vi "Dashboard Main.vi"() -> ()   [LabVIEW 2016]
uses:
  <vilib>/Utility/miscctls.llb/LVRowAndColumnTypeDef.ctl
  <vilib>/event_ctls.llb/eventvkey.ctl
  <vilib>/Rock Robotics/Network Tables/NT Read Numeric Array.vi
  <vilib>/Rock Robotics/Network Tables/NT Read Boolean.vi
  <vilib>/Rock Robotics/WPI/Dashboard/WPI_DashboardLogging Global.vi
panel:
  in  "Camera Settings Right":T1={"Frame Rate"=30, "Compression"=30, "Size"=1, "DB Camera Config"=FALSE} {"Frame Rate" scale=1.0..30.0; "Compression" scale=100.0..-1.0; "Size" items=["640x480", "320x240", "160x120"]}
  out "Camera Info":cluster{"Mbps LED":bool, "Mbps":dbl, "fps":dbl} {"fps" format="%#.1g"; "Mbps" format="%#.1g"}
  in  "Camera Settings":T1={"Frame Rate"=30, "Compression"=30, "Size"=1, "DB Camera Config"=FALSE} {"Frame Rate" scale=1.0..30.0; "Compression" scale=100.0..-1.0; "Size" items=["640x480", "320x240", "160x120"]}
  in  "TCP":refnum<k5>
  in  "Rec Mode":enum32{"Stop", "Record", "Playback"}(radio)
  out "Robot IP":string
  out "Image Message":string="Timeout in Camera Communications"
  in  "Dashboard Tab":T2(tab)
  in  "Select Auto":string(combo)="Select Autonomous ..."
  out "NT Connection":bool
  out "MotorChart R":cluster{"Numeric":dbl, "Numeric":dbl}(graph)
  out "MotorChart L":cluster{"Numeric":dbl, "Numeric":dbl}(graph)
  out "MotorSliders R":cluster{"MotorSlide1":dbl, "MotorSlide2":dbl} {"MotorSlide2" scale=-1.0..1.0 scale format="%#_2e"; "MotorSlide1" scale=-1.0..1.0 scale format="%#_2e"}
  out "MotorSliders L":cluster{"MotorSlide1":dbl, "MotorSlide2":dbl} {"MotorSlide2" scale=-1.0..1.0 scale format="%#_2e"; "MotorSlide1" scale=-1.0..1.0 scale format="%#_2e"}
  out "Gyro":dbl(knob) scale=0.0..360.0
  out "JS1 Z":dbl(slide) scale=-1.0..1.0 scale format="%#_2e"
  out "JS1 Graph":cluster{"X":dbl, "Y":dbl}[](graph)
  out "JS1 Buttons":T3
  out "JS2 Z":dbl(slide) scale=-1.0..1.0 scale format="%#_2e"
  out "JS2 Graph":cluster{"X":dbl, "Y":dbl}[](graph)
  out "JS2 Buttons":T3
  out "Mode":T4(ring)=enum."Auto Disabled"
  out "Camera Image Right":T5(plugin-control)
  in  "ACTION":u16(ring) items=["Place Gear (Default)", "Cross Line Only", "Place Gear And Cross Line"]
  in  "POSITION":dbl format="%#_3f"
  in  "Left":dbl
  in  "Motor":dbl
  in  "Right":dbl
  in  "Camera Name":string(combo)="No Camera Selection"
  out "Scaling Mode":bool
  in  "Camera Name Right":string(combo)="No Camera Selection"
  in  "Test Slider":dbl(slide) scale=0.0..100.0 scale format="%#_3g"
  in  "On/Off":bool caption="Solenoid"
  in  "Test Name":u16(ring) items=["Select the test to run..."]
  in  "Test Tree":string(tree)
  in  "Motor":cluster{"Value":dbl, "Enable":bool} {"Value" scale=-1.0..1.0 scale format="%#_3g"}
  out "Progress":T6 {"Test Progress" scale=0.0..100.0}
  in  "Rev/Fwd":cluster{"Forward":bool, "Reverse":bool}
  in  "Test Ring":u16(ring) items=["Monochrome", "Color"]
  out "Cmd Status":string
  in  "Execute Command":bool
  in  "Command Params":string[][](table)
  in  "Command Selection":i32(listbox)
  in  "CheckList":i32(listbox)
  out "Tree":string(tree)
  out "Camera Image":T5(plugin-control)
  out "Background":bool
  # "HW"
  # "HW"
  # "Joysticks"
  # "Drive Motors"
  # "Front"
  # "Right"
  # "Left"
  # "Back"
  # "AUTONOMOUS- FILL OUT BEFORE EVERY MATCH"
  # "Supply a number between 1 and 3"
  # "Select an action"
  # "Flywheel Speed"
  # "Carousel Motor"
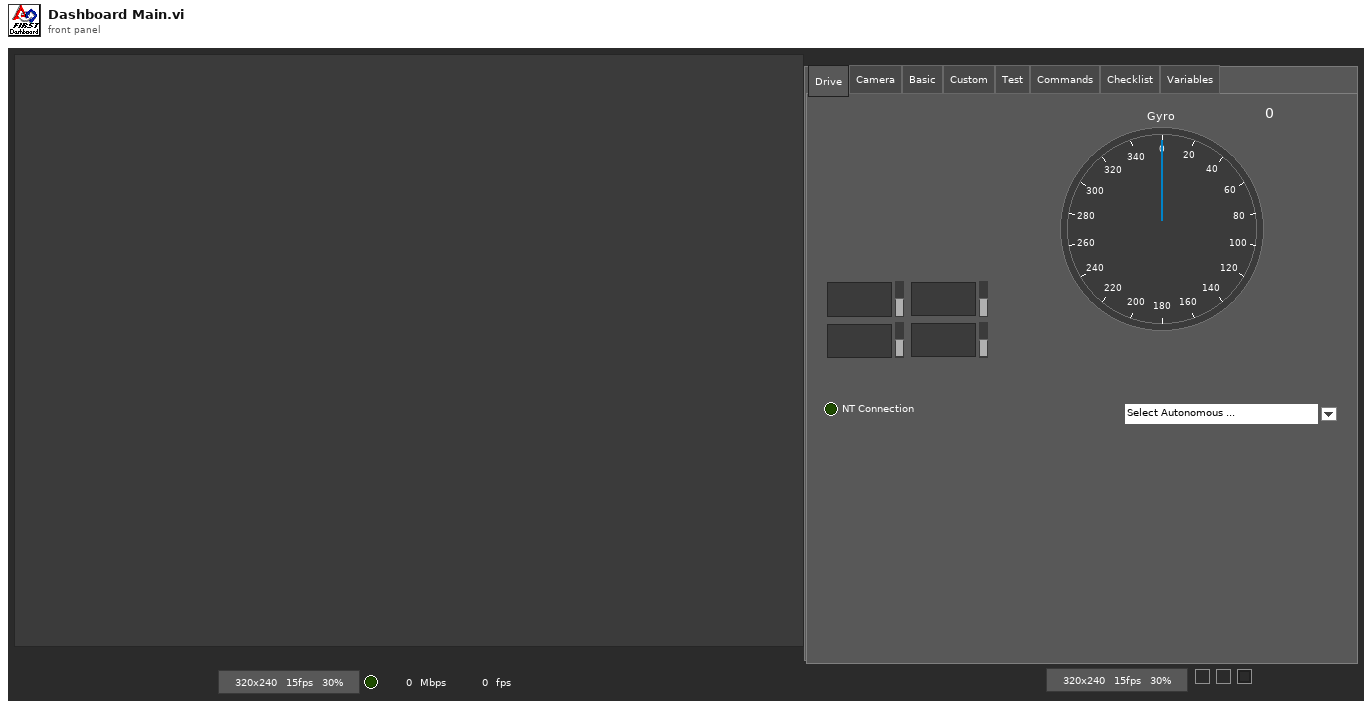
[diagram p1: front panel]
types:
  T1 = cluster{"Frame Rate":i32, "Compression":i32, "Size":u16, "DB Camera Config":bool}
  T2 = enum32{"Drive", "Camera", "Basic", "Custom", "Test", "Commands", "Checklist", "Variables"}
  T3 = cluster{bool, bool, bool, bool, bool, bool, bool, bool, bool, bool, bool, bool}
  T4 = enum8{"Tele-Op Disabled", "Tele-Op Enabled", "Auto Disabled", "Auto Enabled", "Test Disabled", "Test Enabled", "Disconnected", "No Code", "E-Stop"}
  T5 = typedef "IMAQ Image.ctl" = refnum<image>
  T6 = cluster{"Test Progress":u8, "Test Progress Text":string}
  T7 = typedef "Image Type" = u32
  T8 = cluster{"IDs":cluster{"RPC field ID":u16, "Unique ID":u16}, "String":string}
  T9 = enum32{"Drive", "Basic", "Custom", "Test", "Checklist", "Variables"}
  T10 = cluster{"Camera Streams":i32, cluster{"occurrence":refnum<k4>, "New Image":T5}[]}
  T11 = cluster{"Error Strings":string, "Disable Counts":cluster{u16, u16}, "Rail Faults":cluster{u16, u16, u16}, "Robot IP":string, "DB Mode":u8, "Event Info":cluster{"Name":string, "Type":u8, "Number":u16, "Replay":u8}}
  T12 = cluster{"Storage":cluster{"Disk Free":u64, "RAM Block":u32, "RAM free":u32}, "CPU Utilization":cluster{"CPU % ISR":sgl, "CPU % Time Crit":sgl, "CPU % Timed Str":sgl, "CPU % High":sgl, "CPU % Above":sgl, "CPU % Normal":sgl, "CPU % Low":sgl}, "CAN":cluster{"% Bus Utilization":sgl, "Bus Off Cnt":u32, "TX_FIFO Full Cnt":u32, "Receive Error Cnt":u8, "Transmit Error Cnt":u8}, "HID":cluster{"HID Outputs":u32, "Rumble Low":u16, "Rumble High":u16}[]}
  T13 = cluster{"Status bits":cluster{"Test Mode":bool, "Autonomous":bool, "Enabled":bool, "Code Start":bool, "Brownout":bool, "Reserved 2":bool, "Reserved 3":bool, "E-Stop":bool}, "Code Trace":cluster{"Disabled":bool, "TeleOp":bool, "Auto":bool, "Test":bool}, "Controller Type":enum16{"unknown", "cRIO", "roboRio"}, "Code?":enum16{"unknown", "noCode", "code"}, "Battery V":dbl}
  T14 = cluster{"Control Bits":cluster{"TestMode":bool, "Autonomous":bool, "Enabled":bool, "FMS Present":bool, bool, bool, bool, "E-Stop":bool}, "Team Station ":u8, "Countdown":sgl, "Joystick Values":cluster{"Axes":dbl[], "Buttons":bool[], "POVs":i16[]}[]}
  T15 = cluster{"Axes":dbl[], "Buttons":bool[], "POVs":i16[]}[]
  T16 = cluster{"Axes":dbl[], "Buttons":bool[], "POVs":i16[]}
  T17 = cluster{"Buttons[0]":bool, "Buttons[1]":bool, "Buttons[2]":bool, "Buttons[3]":bool, "Buttons[4]":bool, "Buttons[5]":bool, "Buttons[6]":bool, "Buttons[7]":bool, "Buttons[8]":bool, "Buttons[9]":bool, "Buttons[10]":bool, "Buttons[11]":bool}
  T18 = cluster{"Camera Image":refnum<vi>, "Dashboard Tab":refnum<vi>, "Background":refnum<vi>, "Rec Mode":refnum<vi>, "Test Slider":refnum<vi>, "On/Off ":refnum<vi>, "Test Ring":refnum<vi>, "Rev/Fwd":refnum<vi>, "Test Name":refnum<vi>, "Motor":refnum<vi>, "Progress":refnum<vi>, "CheckList":refnum<vi>, "Tree":refnum<vi>, "Test Tree":refnum<vi>, "Command Params":refnum<vi>, "Command Selection":refnum<vi>, "Execute Command":refnum<vi>, "Cmd Status":refnum<vi>, "Camera Settings":refnum<vi>, "Camera Name":refnum<vi>, "Camera Info":refnum<vi>, "Camera Settings Right":refnum<vi>, "Camera Name Right":refnum<vi>, "Camera Image Right":refnum<vi>}
  T19 = cluster{"Operation":enum16{"Update", "Clear"}, "Color Box":u32}[]
  T20 = typedef "eventvkey.ctl" = enum16{"ASCII", "Enter", "Return", "Shift", "Ctrl", "Alt", "Cmd", "Opt", "Caps", "NumLock", "Clear", "Break", "Up", "Down", "Left", "Right", "Insert", "Delete", "Home", "End", "PageUp", "PageDown", "Escape", "Help", "Pause", "ScrollLock", "F1", "F2", "F3", "F4", "F5", "F6", "F7", "F8", "F9", "F10", "F11", "F12", "F13", "F14", "F15", "F16", "F17", "F18", "F19", "F20", "F21", "F22", "F23", "F24", "Play", "VolumeUp", "VolumeDown", "Mute", "Two Byte Char"}
  T21 = cluster{"Image Size":bool, "Image Type":bool, "Pixel Value":bool, "ROI Information":bool, "Zoom Factor":bool}
  T22 = cluster{"Operation":enum16{"Update", "Clear"}, "Color Box":u32}
  T23 = typedef "LVRowAndColumnTypeDef.ctl" = cluster{"Row":i32, "Column":i32}
  T24 = cluster{"Shift":bool, "Ctrl":bool, "Alt":bool, "Cmd":bool, "Opt":bool}
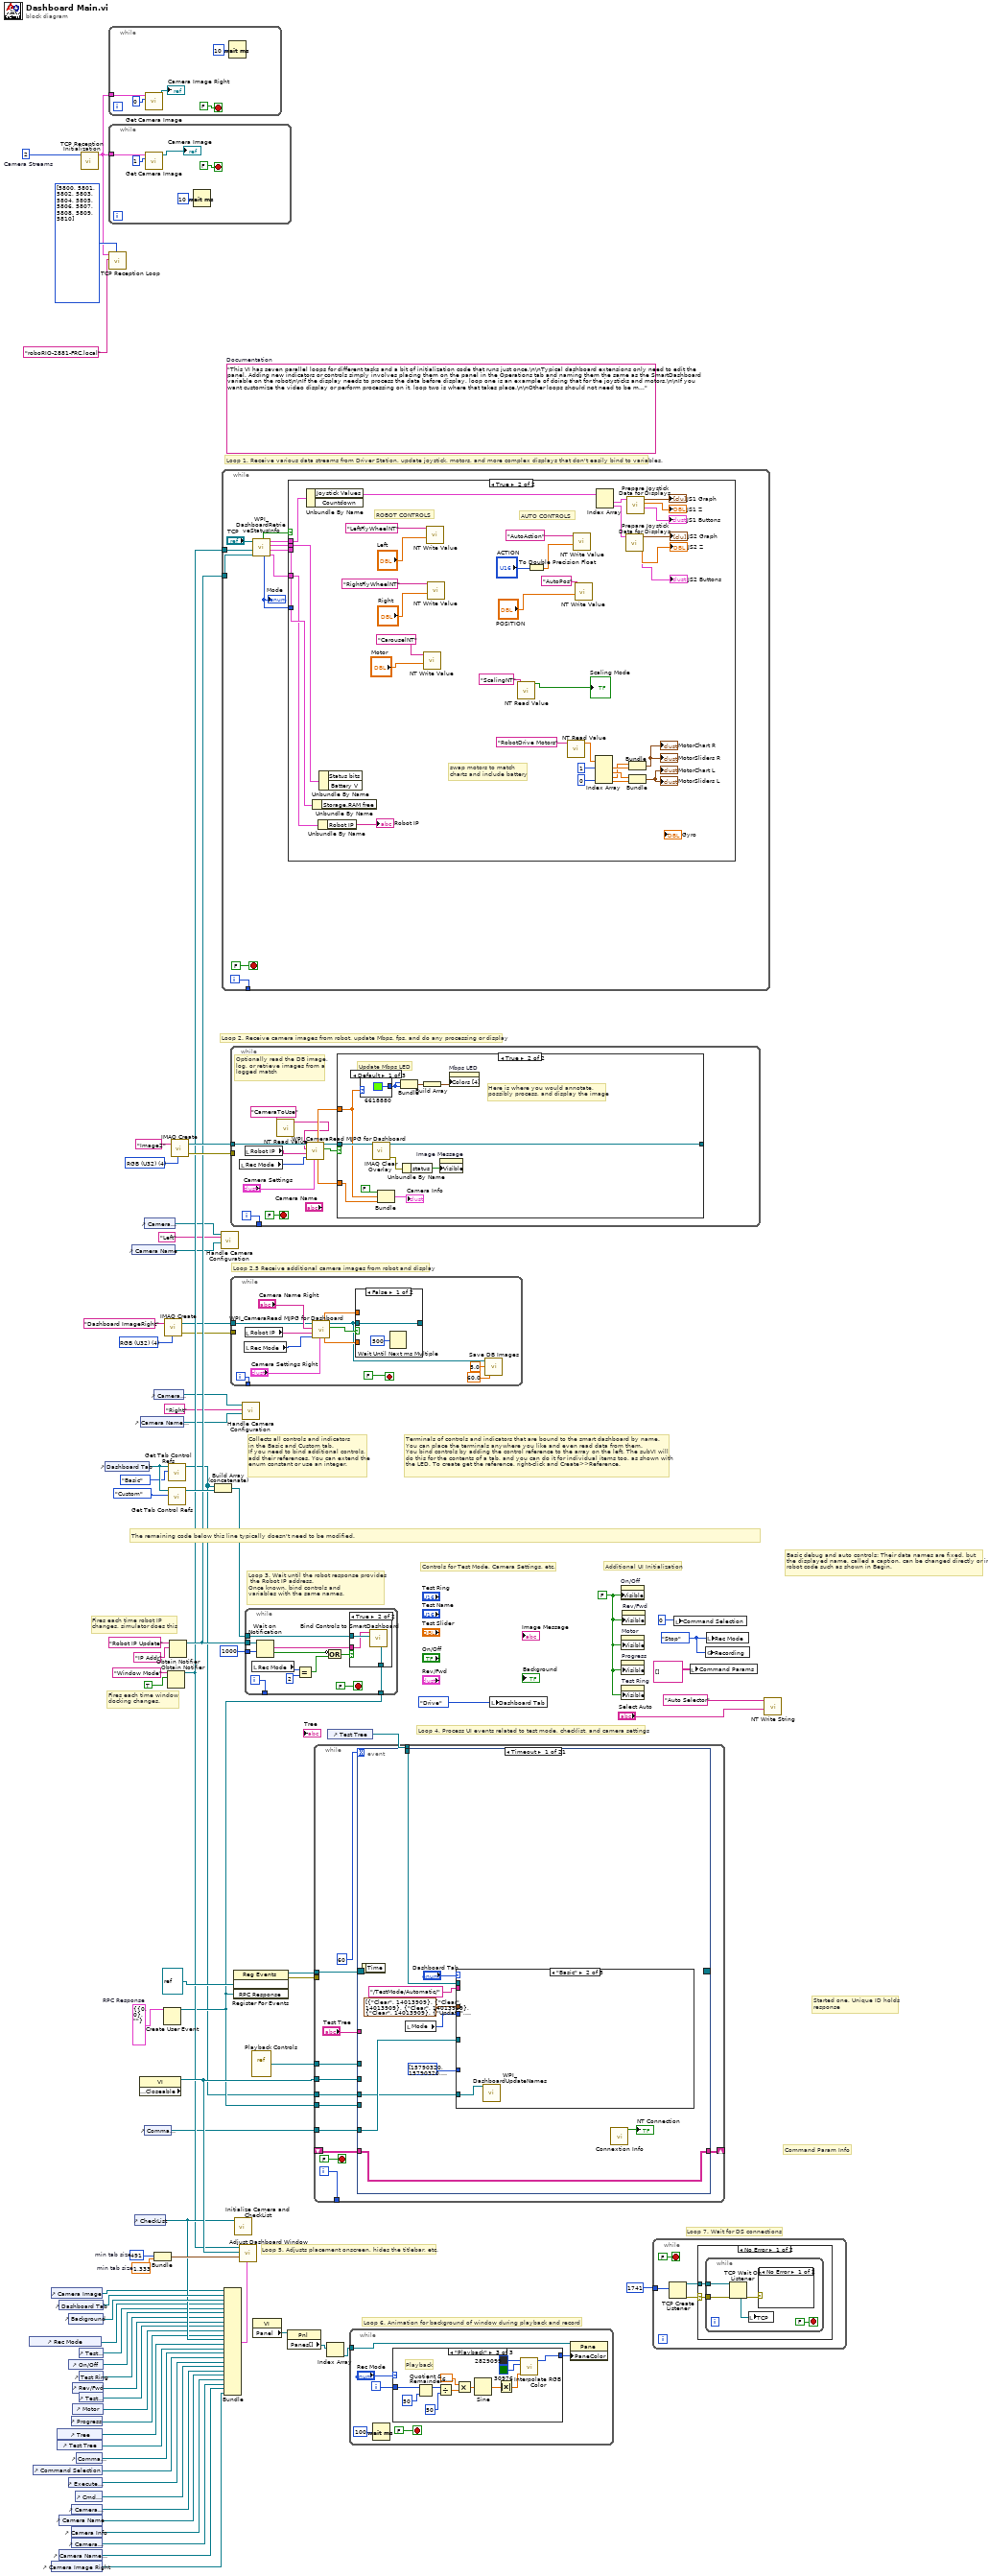
[diagram p0: block diagram]
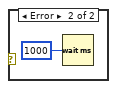
[diagram p3: hidden frame]
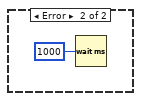
[diagram p4: hidden frame]
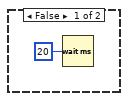
[diagram p5: hidden frame]
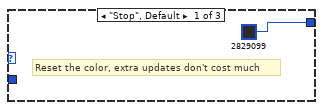
[diagram p6: hidden frame]
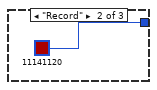
[diagram p7: hidden frame]
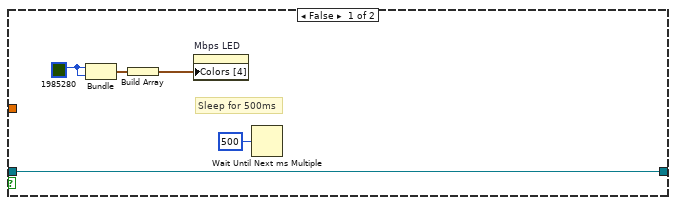
[diagram p9: hidden frame]
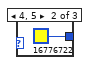
[diagram p10: hidden frame]
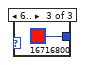
[diagram p11: hidden frame]
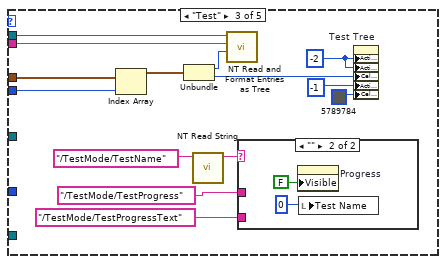
[diagram p13: hidden frame]
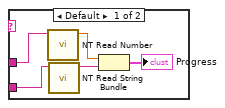
[diagram p14: hidden frame]
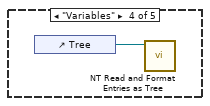
[diagram p15: hidden frame]
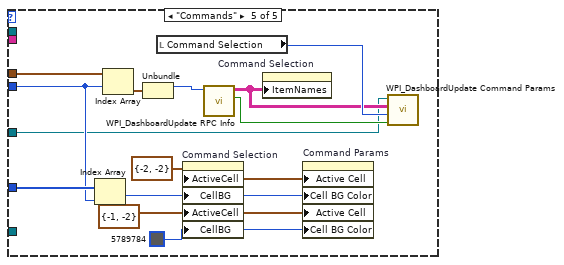
[diagram p16: hidden frame]
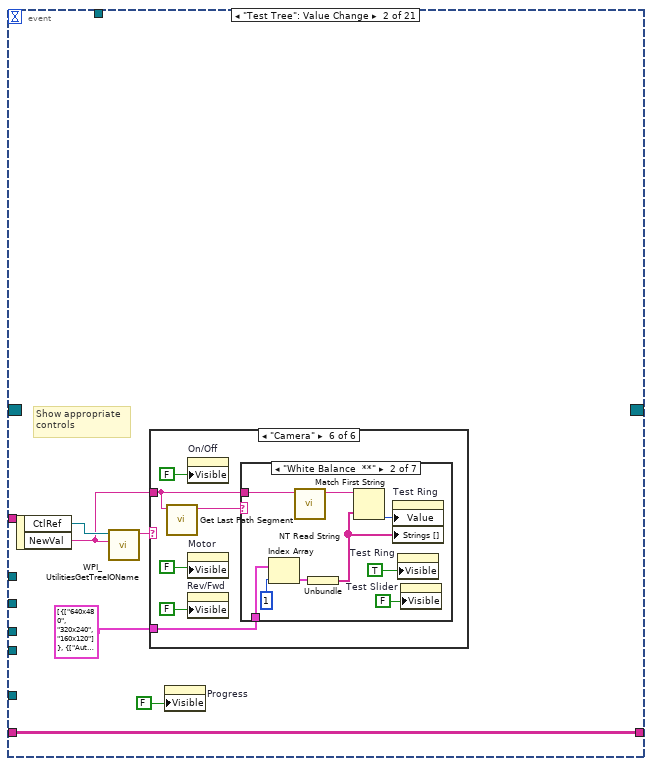
[diagram p17: hidden frame]
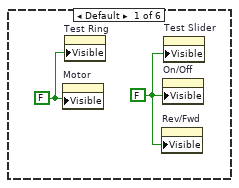
[diagram p18: hidden frame]
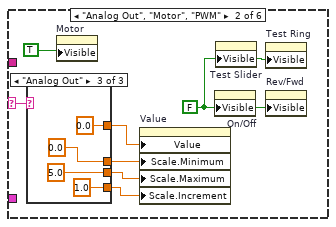
[diagram p19: hidden frame]
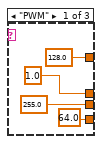
[diagram p20: hidden frame]
diagram:
  w7 = 2  # Camera Streams
  w16 = T7 4 items=["Grayscale (U8)", "Grayscale (I16)", "Grayscale (SGL)", "Complex (CSG)", "RGB (U32)", "HSL (U32)", "RGB (U64)"] ("Image Type")
  w32 = T8 {"IDs"={"RPC field ID"=0, "Unique ID"=0}, "String"=""}  # RPC Response
  w56 = 491  # min tab size
  w55 = 1.333  # min tab size
  w62 = enum32{"Stop", "Record", "Playback"}."Stop" ("Rec Mode")
  w39 = FALSE ("Visible")
  (unwired) "This VI has seven parallel loops for different tasks and a bit of initialization code that runs just once.\n\nTypical dashboard extensions only need to edit the panel. Adding new indicators or controls simply involves placing them on the panel in the Operations tab and naming them the same as the SmartDashboard variable on the robot\n\nIf the display needs to process the data before display, loop one is an example of doing that for the joysticks and motors.\n\nIf you want customize the video display or perform processing on it, loop two is where that takes place.\n\nOther loops should not need to be modified. They are pretty standard, and document the task they perform."  # Documentation
  w79 = T7 4 items=["Grayscale (U8)", "Grayscale (I16)", "Grayscale (SGL)", "Complex (CSG)", "RGB (U32)", "HSL (U32)", "RGB (U64)"] ("Image Type")
  # "Loop 2.5 Receive additional camera images from robot and display"
  # "Command Param Info"
  # "Started one, Unique ID holds\nresponse"
  # "Loop 7. Wait for DS connections"
  # "Basic debug and auto controls: Their data names are fixed, but\nthe displayed name, called a caption, can be changed directly or in\nrobot code such as shown in Begin."
  # "Controls for Test Mode, Camera Settings, etc."
  # "Additional UI Initialization"
  # "Loop 6. Animation for background of window during playback and record"
  # "Fires each time robot IP\nchanges, simulator does this"
  # "Fires each time window\ndocking changes."
  # "Collects all controls and indicators\nin the Basic and Custom tab.\nIf you need to bind additional controls,\nadd their references. You can extend the\nenum constant or use an integer."
  # "The remaining code below this line typically doesn't need to be modified."
  # "Loop 4. Process UI events related to test mode, checklist, and camera settings"
  # "Terminals of controls and indicators that are bound to the smart dashboard by name.\nYou can place the terminals anywhere you like and even read data from them.\nYou bind controls by adding the control reference to the array on the left. The subVI will\ndo this for the contents of a tab, and you can do it for individual items too, as shown with\nthe LED. To create get the reference, right-click and Create>>Reference."
  # "Loop 3. Wait until the robot response provides\n the Robot IP address.\nOnce known, bind controls and\nvariables with the same names."
  # "Loop 5. Adjusts placement onscreen, hides the titlebar, etc."
  # "Loop 1. Receive various data streams from Driver Station, update joystick, motors, and more complex displays that don't easily bind to variables."
  # "Loop 2. Receive camera images from robot, update Mbps, fps, and do any processing or display"
  n1 = control-ref of="Rec Mode"() -> (w45:refnum<vi>)
  n2 = control-ref of="Command Selection"() -> (w31:refnum<vi>)
  n3 = control-ref of="Camera Image Right"() -> (w2:refnum<vi>)
  n4 = control-ref of="Camera Image"() -> (w3:refnum<vi>)
  n5 = control-ref of="Tree"() -> (w49:refnum<vi>)
  n6 = control-ref of="Test Tree"() -> (w48:refnum<vi>)
  n7 = control-ref of="Dashboard Tab"() -> (w57:refnum<vi>)
  n8 = control-ref of="Camera Name"() -> (w22:refnum<vi>)
  n9 = control-ref of="Camera Name Right"() -> (w8:refnum<vi>)
  n10 = control-ref of="Execute Command"() -> (w33:refnum<vi>)
  n11 = control-ref of="Background"() -> (w53:refnum<vi>)
  n12 = control-ref of="On/Off"() -> (w43:refnum<vi>)
  n13 = control-ref of="Progress"() -> (w40:refnum<vi>)
  n14 = control-ref of="Camera Settings"() -> (w23:refnum<vi>)
  n15 = control-ref of="Camera Info"() -> (w21:refnum<vi>)
  n16 = control-ref of="Camera Settings Right"() -> (w9:refnum<vi>)
  n17 = control-ref of="Rev/Fwd"() -> (w41:refnum<vi>)
  n18 = control-ref of="Motor"() -> (w46:refnum<vi>)
  n19 = control-ref of="Cmd Status"() -> (w27:refnum<vi>)
  n20 = control-ref of="Command Params"() -> (w34:refnum<vi>)
  n21 = control-ref of="Test Slider"() -> (w44:refnum<vi>)
  n22 = control-ref of="Test Ring"() -> (w42:refnum<vi>)
  n23 = control-ref of="Test Name"() -> (w47:refnum<vi>)
  n24 = call "TCP Reception Initialization.vi"("Camera Streams"=w7) -> ("Cluster"=w4:T10)  [unwired: 10 in]
  n25 = control-ref of="Dashboard Tab"() -> (w60:refnum<vi>)
  n26 = while {
    tunnel: w4 -> [w82]
    stop <- FALSE stop-if-true
    n27 = call "Get Camera Image.vi"("index"=0, "output cluster"=w82) -> ("Refnum out"=→"Camera Image Right":T5)  [unwired: 9 in]
    n28 = Wait (ms)(milliseconds to wait=u32 10) -> ()  [unwired: 1 out]
  }
  n29 = while {
    tunnel: w4 -> [w87]
    stop <- FALSE stop-if-true
    n30 = call "Get Camera Image.vi"("index"=1, "output cluster"=w87) -> ("Refnum out"=→"Camera Image":T5)  [unwired: 9 in]
    n31 = Wait (ms)(milliseconds to wait=u32 10) -> ()  [unwired: 1 out]
  }
  n32 = call "TCP Reception Loop.vi"("Array 2"=u16[] [5800, 5801, 5802, 5803, 5804, 5805, 5806, 5807, 5808, 5809, 5810], "address"="roboRIO-2881-FRC.local", "output cluster"=w4) -> ()  [unwired: 9 in]
  n33 = control-ref of="Camera Name"() -> (w24:refnum<vi>)
  n34 = control-ref of="CheckList"() -> (w50:refnum<vi>)
  n35 = property class="VI" props=["Front Panel.Closeable"]() -> (reference out=w61:refnum<vi>)  [unwired: 2 in, 2 out]
  n36 = control-ref of="Camera Name Right"() -> (w12:refnum<vi>)
  n37 = control-ref of="Camera Settings"() -> (w25:refnum<vi>)
  n38 = control-ref of="Command Params"() -> (w26:refnum<vi>)
  n39 = control-ref of="Camera Settings Right"() -> (w13:refnum<vi>)
  n40 = Bundle("min tab size"=w56, "min tab size"=w55) -> (w54:cluster{"min tab size":i32, "min tab size":dbl})  [unwired: 1 in]
  n41 = Create User Event(user event datatype=w32) -> (user event=w28:refnum<user-event>)  [unwired: 1 in, 1 out]
  n42 = call "IMAQ Create"("Image Name"="Dashboard ImageRight", "Image Type"=w16) -> ("New Image"=w15:T5, "error out"=w14:errorcluster)  [unwired: 2 in, 1 out]
  n43 = Obtain Notifier(name (unnamed)="Window Mode", notification data type=TRUE) -> (notifier out=w37:refnum<notifier>)  [unwired: 2 in, 2 out]
  n44 = call <vilib>:"Get Tab Control Refs.vi"("Page Index"=T9."Basic" ("Dashboard Tab"), "TabControl in"=w60) -> ("ControlsOnPage"=w20:refnum<vi>[])  [unwired: 9 in]
  n45 = call <vilib>:"Get Tab Control Refs.vi"("Page Index"=T9."Custom" ("Dashboard Tab"), "TabControl in"=w60) -> ("ControlsOnPage"=w59:refnum<vi>[])  [unwired: 9 in]
  n46 = Obtain Notifier(name (unnamed)="Robot IP Update", notification data type="IP Addr" ("name (unnamed)")) -> (notifier out=w38:refnum<notifier>)  [unwired: 2 in, 2 out]
  n47 = call "IMAQ Create"("Image Name"="Image2", "Image Type"=w79) -> ("New Image"=w77:T5, "error out"=w76:errorcluster)  [unwired: 2 in, 1 out]
  n48 = Build Array (concatenate)(w20, w59) -> (w58:refnum<vi>[])
  n49 = call "Handle Camera Configuration.vi"("CameraNameRef"=w24, "Camera File Name"="Left", "ClusterRef"=w25) -> ()  [unwired: 9 in]
  n50 = while {
    tunnel: [w99] -> _
    tunnel: w38 -> [w93]
    tunnel: w37 -> [w90]
    i -> [w99]
    stop <- FALSE stop-if-true
    n51 = call <vilib>:"WPI_DashboardRetrieveStatusInfo.vi"("Binding Refnum"=w93, "Window Mode Notifier"=w90, "TCP Cnx"="TCP") -> ("Power and Errors"=w94:T11, "Robot Metrics"=w97:T12, "Status Info"=w98:T13, "Control Info"=w95:T14, "Robot Mode"=w92:T4, "Process?"=w96:bool)  [unwired: 3 in]
    "Mode" <- w92
    n52 = case shown="True" w96 {
      tunnel: w98 -> [_ w138]
      tunnel: w97 -> [_ w137]
      tunnel: w95 -> [_ w136]
      tunnel: w94 -> [_ w135]
      tunnel: w92 -> [_ _]
      frame False {
        n53 = Wait (ms)(milliseconds to wait=u32 20) -> ()  [unwired: 1 out]
      }
      frame True {
        # "AUTO CONTROLS"
        # "ROBOT CONTROLS"
        # "swap motors to match\ncharts and include battery"
        n54 = Unbundle By Name(w136) -> ("Joystick Values"=w126:T15)  [unwired: 1 out]
        n55 = Unbundle By Name(w137) -> ()  [unwired: 1 out]
        n56 = Unbundle By Name(w135) -> ("Robot IP"=→"Robot IP":string)
        n57 = Unbundle By Name(w138) -> ()  [unwired: 2 out]
        n58 = call-poly <vilib>:"NT Write Value.vi"("Numeric"="Motor", "Name"="CarouselNT") -> ()  [unwired: 9 in, 1 out]
        n59 = call-poly <vilib>:"NT Write Value.vi"("Numeric"="Left", "Name"="LeftFlyWheelNT") -> ()  [unwired: 9 in, 1 out]
        n60 = call-poly <vilib>:"NT Write Value.vi"("Numeric"="Right", "Name"="RightFlyWheelNT") -> ()  [unwired: 9 in, 1 out]
        n61 = call-poly <vilib>:"NT Read Value.vi"("Name"="ScalingNT") -> ("Boolean"=→"Scaling Mode":bool)  [unwired: 9 in, 1 out]
        n62 = To Double Precision Float(number="ACTION") -> (double precision float=w107:dbl)
        n63 = call-poly <vilib>:"NT Read Value.vi"("Name"="RobotDrive Motors") -> ("Numeric Array"=w116:dbl[])  [unwired: 9 in, 1 out]
        n64 = call-poly <vilib>:"NT Write Value.vi"("Numeric"=w107, "Name"="AutoAction") -> ()  [unwired: 9 in, 1 out]
        n65 = call-poly <vilib>:"NT Write Value.vi"("Numeric"="POSITION", "Name"="AutoPos") -> ()  [unwired: 9 in, 1 out]
        n66 = Index Array(array=w116, index #1=1, index #4=0) -> (element #1=w130:dbl, element #2=w131:dbl, element #3=w129:dbl, element #4=w134:dbl)  [unwired: 2 in]
        n67 = Index Array(array=w126) -> (element #1=w125:T16, element #2=w121:T16)  [unwired: 2 in]
        n68 = call "Prepare Joystick Data for Displays.vi"("Joystick Values"=w121) -> ("Buttons"=→"JS2 Buttons":T17, "Z Axis"=→"JS2 Z":dbl, "Cartesian Data"=→"JS2 Graph":cluster{"X axis":dbl, "X axis":dbl}[])  [unwired: 8 in]
        n69 = call "Prepare Joystick Data for Displays.vi"("Joystick Values"=w125) -> ("Buttons"=→"JS1 Buttons":T17, "Z Axis"=→"JS1 Z":dbl, "Cartesian Data"=→"JS1 Graph":cluster{"X axis":dbl, "X axis":dbl}[])  [unwired: 8 in]
        n70 = Bundle("Numeric"=w129, "Numeric"=w130) -> (→"MotorChart R" →"MotorSliders R":cluster{"Numeric":dbl, "Numeric":dbl})  [unwired: 1 in]
        n71 = Bundle("Numeric"=w131, "Numeric"=w134) -> (→"MotorChart L" →"MotorSliders L":cluster{"Numeric":dbl, "Numeric":dbl})  [unwired: 1 in]
      }
    }
  }
  n72 = Bundle("Camera Image"=w3, "Dashboard Tab"=w57, "Background"=w53, "Rec Mode"=w45, "Test Slider"=w44, "On/Off"=w43, "Test Ring"=w42, "Rev/Fwd"=w41, "Test Name"=w47, "Motor"=w46, "Progress"=w40, "CheckList"=w50, "Tree"=w49, "Test Tree"=w48, "Command Params"=w34, "Command Selection"=w31, "Execute Command"=w33, "Cmd Status"=w27, "Camera Settings"=w23, "Camera Name"=w22, "Camera Info"=w21, "Camera Settings Right"=w9, "Camera Name Right"=w8, "Camera Image Right"=w2) -> (w1:T18)  [unwired: 1 in]
  n73 = while {
    tunnel: w77 -> [w148]
    tunnel: w76 -> [_]
    tunnel: [w149] -> _
    i -> [w149]
    stop <- FALSE stop-if-true
    # "Optionally read the DB image,\nlog, or retrieve images from a\nlogged match"
    n74 = local read "Rec Mode"() -> (w144:enum32{"Stop", "Record", "Playback"})
    n75 = local read "Robot IP"() -> (w143:string)
    n76 = call-poly <vilib>:"NT Read Value.vi"("Name"="CameraToUse") -> ("String"=w139:string)  [unwired: 9 in, 1 out]
    n77 = call <vilib>:"WPI_CameraRead MJPG for Dashboard.vi"("Camera Settings"="Camera Settings", "Rec Mode"=w144, "Robot IP"=w143, "Camera Name"=w139, "Refnum in"=w148) -> ("Active"=w146:bool, "Refnum out"=w147:T5, "FPS"=w145:dbl, "Bandwidth (Mbps)"=w142:dbl)  [unwired: 3 in]
    n78 = case shown="True" w146 {
      tunnel: w147 -> [w151 w162]
      tunnel: w142 -> [_ w159]
      tunnel: w145 -> [_ w160]
      tunnel: [w151 w156] -> _
      frame False {
        w153 = u32 1985280 ("Color Box")
        # "Sleep for 500ms"
        n79 = Bundle("Color Box"=w153, "Color Box"=w153) -> (w154:cluster{"Color Box":u32, "Color Box":u32})  [unwired: 1 out]
        n80 = Build Array(w154) -> (w152:cluster{"Color Box":u32, "Color Box":u32}[])
        n81 = property on="Mbps LED" class="Bool (strict)"("Colors [4]"=w152) -> ()  [unwired: 2 in, 2 out]
        n82 = Wait Until Next ms Multiple(millisecond multiple=u32 500) -> ()  [unwired: 1 out]
      }
      frame True {
        # "Here is where you would annotate,\npossibly process, and display the image"
        # "Update Mbps LED"
        n83 = case shown="Default" w159 {
          tunnel: [u32 6618880 ("Color Box") u32 16776722 ("Color Box") u32 16716800 ("Color Box")] -> w163
          frame Default {
          }
          frame 4, 5 {
          }
          frame 6.. {
          }
        }
        n84 = call "IMAQ Clear Overlay"("Image"=w162) -> ("error out"=w165:errorcluster, "Image Out"=w156:T5)  [unwired: 2 in, 7 out]
        n85 = Bundle(FALSE, "Bandwidth (Mbps)"=w159, "FPS"=w160) -> (→"Camera Info":cluster{bool, "Bandwidth (Mbps)":dbl, "FPS":dbl})  [unwired: 1 in]
        n86 = Bundle("Color Box"=w163, "Color Box"=w163) -> (w164:cluster{"Color Box":u32, "Color Box":u32})  [unwired: 1 out]
        n87 = Unbundle By Name(w165) -> ("status"=w166:bool)
        n88 = Build Array(w164) -> (w161:cluster{"Color Box":u32, "Color Box":u32}[])
        n89 = property on="Image Message" class="Str"("Visible"=w166) -> ()  [unwired: 2 in, 2 out]
        n90 = property on="Mbps LED" class="Bool (strict)"("Colors [4]"=w161) -> ()  [unwired: 2 in, 2 out]
      }
    }
  }
  n91 = while {
    tunnel: w15 -> [w181]
    tunnel: w14 -> [_]
    tunnel: [w176] -> _
    i -> [w176]
    stop <- FALSE stop-if-true
    n92 = local read "Rec Mode"() -> (w179:enum32{"Stop", "Record", "Playback"})
    n93 = local read "Robot IP"() -> (w180:string)
    n94 = call <vilib>:"WPI_CameraRead MJPG for Dashboard.vi"("Camera Settings"="Camera Settings Right", "Rec Mode"=w179, "Robot IP"=w180, "Camera Name"="Camera Name Right", "Refnum in"=w181) -> ("Active"=w175:bool, "Refnum out"=w172:T5, "FPS"=w173:dbl, "Bandwidth (Mbps)"=w174:dbl)  [unwired: 3 in]
    n95 = case shown="False" w175 {
      tunnel: w172 -> [w183 w185]
      tunnel: w174 -> [_ _]
      tunnel: w173 -> [_ _]
      tunnel: [w183 w185] -> _
      frame False {
        n96 = Wait Until Next ms Multiple(millisecond multiple=u32 500) -> ()  [unwired: 1 out]
      }
      frame True {
      }
    }
    n97 = call "Save DB Images.vi"("Images to Keep"=60.0, "Time Interval (s)"=5.0, "Image"=w172) -> ()  [unwired: 1 in]
  }
  n98 = register-events(refnum<vi> refnum, w28) -> (reference out=w66:refnum<event-registration>, error out=w65:errorcluster)  [unwired: 2 in]
  n99 = call "Initialize Camera and CheckList.vi"("ListBox in"=w50) -> ()  [unwired: 11 in]
  n100 = call "Adjust Dashboard Window.vi"("Sizing Refnums"=w1, "Size Constraints"=w54, "VI"=w61, "WIn Mode"=w37) -> ()  [unwired: 8 in]
  n101 = call "Handle Camera Configuration.vi"("CameraNameRef"=w12, "Camera File Name"="Right", "ClusterRef"=w13) -> ()  [unwired: 9 in]
  n102 = while {
    tunnel: w58 -> [w197]
    tunnel: w38 -> [w195]
    tunnel: [w193] -> _
    tunnel: u32 1000 ("milliseconds to wait") -> [w192]
    tunnel: w28 -> [w186]
    i -> [w193]
    stop <- FALSE stop-if-true
    n103 = local read "Rec Mode"() -> (w188:enum32{"Stop", "Record", "Playback"})
    n104 = Wait on Notification(notifier=w195, timeout in ms (-1)=w192) -> (notification=w194:string, timed out?=w190:bool)  [unwired: 2 in, 2 out]
    n105 = Equal?(x=w188, y=u16 2 ("Rec Mode")) -> (x = y?=w189:bool)
    n106 = Compound Arithmetic op=OR(invert w190, w189) -> (w191:bool)
    n107 = case shown="True" w191 {
      tunnel: w197 -> [_ w200]
      tunnel: w194 -> [_ w199]
      tunnel: w186 -> [_ w198]
      frame False {
      }
      frame True {
        n108 = call <vilib>:"Bind Controls to SmartDashboard.vi"("RPC ref"=w198, "Bound Control Refs"=w200, "Server IP Address"=w199) -> ()  [unwired: 9 in]
      }
    }
  }
  n109 = vi-ref "Playback Controls.vi"() -> (w67:refnum<vi>)
  n110 = property class="VI"() -> ("Panel"=w69:refnum<vi>)  [unwired: 2 in, 2 out]
  n111 = property class="Pnl"(reference=w69) -> ("Panes[]"=w70:refnum<vi>[])  [unwired: 1 in, 2 out]
  n112 = Index Array(array=w70) -> (element=w68:refnum<vi>)  [unwired: 1 in]
  n113 = control-ref of="Test Tree"() -> (w71:refnum<vi>)
  n114 = while {
    tunnel: [w210] -> _
    tunnel: w71 -> [w209]
    tunnel: w67 -> [w208]
    tunnel: w66 -> [w207]
    tunnel: w65 -> [_]
    tunnel: w61 -> [w206]
    tunnel: w28 -> [w205]
    tunnel: w26 -> [w204]
    shift-right: [w203] -> _
    shift-left: _ -> [w202]
    tunnel: w20 -> [w201]
    i -> [w210]
    stop <- FALSE stop-if-true
    n115 = event shown="[0] Timeout" {
      selector: w207 -> [_ _ _ _ _ _ _ _ _ _ _ _ _ _ _ _ _ _ _ _ _]
      dyn-events: [_ _ _ _ _ _ _ _ _ _ _ _ _ _ _ _ w466 _ _ _ _] -> _
      timeout: u32 60 ("milliseconds to wait") -> [_ _ _ _ _ _ _ _ _ _ _ _ _ _ _ _ _ _ _ _ _]
      tunnel: w209 -> [w222 _ _ _ _ _ _ _ _ _ _ _ _ _ _ _ _ _ _ _ _]
      tunnel: "Test Tree" -> [_ _ _ _ _ _ _ _ _ _ _ w433 w441 w443 w447 w455 _ _ _ _ _]
      tunnel: w208 -> [_ _ _ _ _ _ _ _ _ _ _ _ _ _ _ _ w468 _ w486 _ _]
      tunnel: w206 -> [_ _ _ _ _ _ _ _ _ _ _ _ _ _ _ _ w464 _ _ _ _]
      tunnel: w205 -> [_ _ _ _ _ _ _ _ _ _ _ _ _ _ _ _ w460 _ _ _ _]
      tunnel: w204 -> [w217 _ _ _ _ _ w384 _ _ _ _ _ _ _ _ _ _ _ _ _ _]
      tunnel: [w216 w261 w363 w368 w377 w381 w382 w391 w401 w408 w420 w432 w439 w442 w446 w454 w459 w481 w483 w487 w498] -> w203
      tunnel: w202 -> [w216 w261 w363 w368 w377 w381 w382 _ _ w408 w420 w432 w439 w442 w446 w454 w459 w481 w483 w487 w498]
      tunnel: w201 -> [w214 _ _ _ _ _ _ _ _ _ _ _ _ _ _ _ _ _ _ _ _]
      event Timeout {
        n116 = event-data() -> ()  [unwired: 1 in, 1 out]
        n117 = local read "Mode"() -> (w219:T4)
        n118 = case shown="\"Basic\"" "Dashboard Tab" {
          tunnel: w222 -> [_ _ w238 _ _]
          tunnel: "/TestMode/Automatic/" ("Name Pattern") -> [_ _ w237 _ _]
          tunnel: T19 [{"Operation"=enum."Clear", "Color Box"=14013909}, {"Operation"=enum."Clear", "Color Box"=14013909}, {"Operation"=enum."Clear", "Color Box"=14013909}, {"Operation"=enum."Clear", "Color Box"=14013909}, {"Operation"=enum."Update", "Color Box"=14013909}, {"Operation"=enum."Update", "Color Box"=16777215}, {"Operation"=enum."Clear", "Color Box"=14013909}, {"Operation"=enum."Clear", "Color Box"=14013909}, {"Operation"=enum."Clear", "Color Box"=14013909}] -> [_ _ w230 _ w254]
          tunnel: w219 -> [_ _ w229 _ w253]
          tunnel: u32[] [15790320, 15790320, 15790320, 15790320, 16777215, 16777215, 15790320, 15790320, 15790320] -> [_ _ _ _ w259]
          tunnel: w217 -> [_ _ _ _ w247]
          tunnel: w214 -> [_ w224 _ _ _]
          frame "Custom", Default {
          }
          frame "Basic" {
            n119 = call <vilib>:"WPI_DashboardUpdateNames.vi"("Controls on Tab"=w224) -> ()  [unwired: 11 in]
          }
          frame "Test" {
            w236 = -2 ("Active Item:Row Number")
            n120 = Index Array(array=w230, index=w229) -> (element=w231:T22)
            n121 = Unbundle(w231) -> ("Operation"=w232:enum16{"Update", "Clear"}, "Color Box"=w233:u32)
            n122 = call <vilib>:"NT Read String.vi"("Name"="/TestMode/TestName") -> ("String"=w227:string)  [unwired: 9 in, 1 out]
            n123 = call <vilib>:"NT Read and Format Entries as Tree.vi"("Operation"=w232, "Name Pattern"=w237, "Tree Refnum"=w238) -> ()  [unwired: 7 in, 2 out]
            n124 = case shown="\"\"" w227 {
              tunnel: "/TestMode/TestProgress" ("Name") -> [w240 _]
              tunnel: "/TestMode/TestProgressText" ("Name") -> [w239 _]
              frame Default {
                n125 = call <vilib>:"NT Read Number.vi"("Name"=w240) -> ("Numeric"=w241:dbl)  [unwired: 9 in, 1 out]
                n126 = call <vilib>:"NT Read String.vi"("Name"=w239) -> ("String"=w242:string)  [unwired: 9 in, 1 out]
                n127 = Bundle("Numeric"=w241, "String"=w242) -> (→"Progress":cluster{"Numeric":dbl, "String":string})  [unwired: 1 in]
              }
              frame "" {
                n128 = property on="Progress" class="Clust (strict)"("Visible"=FALSE) -> ()  [unwired: 2 in, 2 out]
                n129 = local write "Test Name"(u16 0) -> ()
              }
            }
            n130 = property on="Test Tree" class="Tree (strict)"("Active Item Row Number"=w236, "ActiveColNum"=w236, "CellBG"=w233, "Active Item Row Number"=-1 ("Active Item:Row Number"), "CellBG"=u32 5789784 ("Color Box")) -> ()  [unwired: 2 in, 2 out]
          }
          frame "Variables" {
            n131 = control-ref of="Tree"() -> (w246:refnum<vi>)
            n132 = call <vilib>:"NT Read and Format Entries as Tree.vi"("Tree Refnum"=w246) -> ()  [unwired: 9 in, 2 out]
          }
          frame "Commands" {
            w255 = u32 5789784 ("Color Box")
            w256 = T23 {"Row"=-1, "Column"=-2} ("Active Cell:Active Cell")
            w258 = T23 {"Row"=-2, "Column"=-2} ("Active Cell:Active Cell")
            n133 = Index Array(array=w259, index=w253) -> (element=w257:u32)
            n134 = Index Array(array=w254, index=w253) -> (element=w252:T22)
            n135 = Unbundle(w252) -> ("Operation"=w251:enum16{"Update", "Clear"})  [unwired: 1 out]
            n136 = local read "Command Selection"() -> (w250:i32)
            n137 = property on="Command Selection" class="MCListbox (strict)"("ActiveCell"=w258, "CellBG"=w257, "ActiveCell"=w256, "CellBG"=w255) -> ()  [unwired: 2 in, 2 out]
            n138 = call <vilib>:"WPI_DashboardUpdate RPC Info.vi"("Operation"=w251) -> ("update"=w249:bool, "commands"=w248:string[][])  [unwired: 9 in]
            n139 = property on="Command Selection" class="MCListbox (strict)"("ItemNames"=w248) -> ()  [unwired: 2 in, 2 out]
            n140 = property on="Command Params" class="Tbl (strict)"("Active Cell"=w258, "Cell BG Color"=w257, "Active Cell"=w256, "Cell BG Color"=w255) -> ()  [unwired: 2 in, 2 out]
            n141 = call <vilib>:"WPI_DashboardUpdate Command Params.vi"("Update"=w249, "NewVal"=w250, "Commands"=w248, "Param Tbl"=w247) -> ()  [unwired: 7 in, 1 out]
          }
        }
        n142 = call <vilib>:"Connextion Info.vi"() -> ("Connected"=→"NT Connection":bool)  [unwired: 10 in, 1 out]
      }
      event "Test Tree": Value Change {
        # "Show appropriate\ncontrols"
        n143 = event-data() -> ("CtlRef"=w264:refnum<vi>, "NewVal"=w262:string)  [unwired: 1 in]
        n144 = call <vilib>:"WPI_UtilitiesGetTreeIOName.vi"("NewVal"=w262, "TreeControl in"=w264) -> ("I/O Name"=w265:string)  [unwired: 9 in]
        n145 = case shown="\"Camera\"" w265 {
          selector: w265 -> [_ w272 _ w294 w303 _]
          tunnel: w262 -> [_ _ w291 w293 _ w310]
          tunnel: cluster{string[]}[] [{["640x480", "320x240", "160x120"]}, {["Auto", "Fixed indoor", "Fixed outdoor 1", "Fixed outdoor 2", "Fixed fluorescent 1", "Fixed fluorescent 2", "Hold current"]}, {["Auto", "Flicker-free 50 Hz", "Flicker-free 60 Hz", "Hold current"]}, {["None", "Prioritize frame rate", "Prioritize image quality"]}, {["Monochrome", "Color"]}] -> [_ _ _ _ _ w309]
          frame Default {
            w267 = FALSE ("Visible")
            w266 = FALSE ("Visible")
            n146 = property on="Motor" class="Clust (strict)"("Visible"=w266) -> ()  [unwired: 2 in, 2 out]
            n147 = property on="Test Ring" class="Ring (strict)"("Visible"=w266) -> ()  [unwired: 2 in, 2 out]
            n148 = property on="Rev/Fwd" class="Clust (strict)"("Visible"=w267) -> ()  [unwired: 2 in, 2 out]
            n149 = property on="On/Off" class="Bool (strict)"("Visible"=w267) -> ()  [unwired: 2 in, 2 out]
            n150 = property on="Test Slider" class="Slide (strict)"("Visible"=w267) -> ()  [unwired: 2 in, 2 out]
          }
          frame "Analog Out", "Motor", "PWM" {
            w273 = FALSE ("Visible")
            n151 = case shown="\"Analog Out\"" w272 {
              tunnel: [1.0 ("Value") -1.0 ("Value") 0.0 ("Value")] -> w271
              tunnel: [255.0 ("Value") 1.0 ("Value") 5.0 ("Value")] -> w270
              tunnel: [128.0 ("Value") 0.0 ("Value") 0.0 ("Value")] -> w269
              tunnel: [64.0 ("Value") 0.5 ("Value") 1.0 ("Value")] -> w268
              frame "PWM" {
              }
              frame "Motor", Default {
              }
              frame "Analog Out" {
              }
            }
            n152 = property on="Motor" class="Clust (strict)"("Visible"=TRUE) -> ()  [unwired: 2 in, 2 out]
            n153 = property on="Value" class="Slide (strict)"("Value"=w269, "Scale.Minimum"=w271, "Scale.Maximum"=w270, "Scale.Increment"=w268) -> ()  [unwired: 2 in, 2 out]
            n154 = property on="On/Off" class="Bool (strict)"("Visible"=w273) -> ()  [unwired: 2 in, 2 out]
            n155 = property on="Test Slider" class="Slide (strict)"("Visible"=w273) -> ()  [unwired: 2 in, 2 out]
            n156 = property on="Test Ring" class="Ring (strict)"("Visible"=w273) -> ()  [unwired: 2 in, 2 out]
            n157 = property on="Rev/Fwd" class="Clust (strict)"("Visible"=w273) -> ()  [unwired: 2 in, 2 out]
          }
          frame "Servo" {
            w289 = FALSE ("Visible")
            n158 = call <vilib>:"NT Read Number.vi"("Name"=w291) -> ("Numeric"=w290:dbl)  [unwired: 9 in, 1 out]
            n159 = property on="Test Slider" class="Slide (strict)"("Visible"=TRUE, "Scale.Maximum"=170.0 ("Scale.Range:Maximum")) -> ()  [unwired: 2 in, 2 out]
            n160 = local write "Test Slider"(w290) -> ()
            n161 = property on="Motor" class="Clust (strict)"("Visible"=w289) -> ()  [unwired: 2 in, 2 out]
            n162 = property on="Rev/Fwd" class="Clust (strict)"("Visible"=w289) -> ()  [unwired: 2 in, 2 out]
            n163 = property on="On/Off" class="Bool (strict)"("Visible"=w289) -> ()  [unwired: 2 in, 2 out]
            n164 = property on="Test Ring" class="Ring (strict)"("Visible"=w289) -> ()  [unwired: 2 in, 2 out]
          }
          frame "Relay", "Solenoid" {
            w292 = FALSE ("Visible")
            n165 = property on="Motor" class="Clust (strict)"("Visible"=w292) -> ()  [unwired: 2 in, 2 out]
            n166 = property on="Test Slider" class="Slide (strict)"("Visible"=w292) -> ()  [unwired: 2 in, 2 out]
            n167 = Search and Replace String(input string=w293, search string="/Value  **", replace string="/Direction") -> (result string=w299:string)  [unwired: 5 in, 3 out]
            n168 = property on="Test Ring" class="Ring (strict)"("Visible"=w292) -> ()  [unwired: 2 in, 2 out]
            n169 = call <vilib>:"NT Read String.vi"("Name"=w299) -> ("String"=w297:string)  [unwired: 9 in, 1 out]
            n170 = Equal?(x="Both directions", y=w297) -> (x = y?=w295:bool)
            n171 = Not(x=w295) -> (.not. x?=w296:bool)
            n172 = property on="Rev/Fwd" class="Clust (strict)"("Visible"=w295) -> ()  [unwired: 2 in, 2 out]
            n173 = property on="On/Off" class="Bool (strict)"("Visible"=w296, "Caption.Text"=w294) -> ()  [unwired: 2 in, 2 out]
          }
          frame "Compressor", "Digital Out" {
            w302 = FALSE ("Visible")
            # "Get direction and finish"
            n174 = property on="Motor" class="Clust (strict)"("Visible"=w302) -> ()  [unwired: 2 in, 2 out]
            n175 = property on="Test Slider" class="Slide (strict)"("Visible"=w302) -> ()  [unwired: 2 in, 2 out]
            n176 = property on="Test Ring" class="Ring (strict)"("Visible"=w302) -> ()  [unwired: 2 in, 2 out]
            n177 = property on="On/Off" class="Bool (strict)"("Visible"=TRUE, "Caption.Text"=w303) -> ()  [unwired: 2 in, 2 out]
            n178 = property on="Rev/Fwd" class="Clust (strict)"("Visible"=FALSE) -> ()  [unwired: 2 in, 2 out]
          }
          frame "Camera" {
            n179 = call <vilib>:"Get Last Path Segment.vi"("String in"=w310) -> ("String out"=w311:string)  [unwired: 10 in]
            n180 = property on="On/Off" class="Bool (strict)"("Visible"=FALSE) -> ()  [unwired: 2 in, 2 out]
            n181 = property on="Motor" class="Clust (strict)"("Visible"=FALSE) -> ()  [unwired: 2 in, 2 out]
            n182 = property on="Rev/Fwd" class="Clust (strict)"("Visible"=FALSE) -> ()  [unwired: 2 in, 2 out]
            n183 = case shown="\"White Balance  **\"" w311 {
              tunnel: w310 -> [w317 w326 w335 w344 w353 _ w359]
              tunnel: w309 -> [w315 w323 w332 w341 w350 _ _]
              frame "Size  **" {
                n184 = Index Array(array=w315) -> (element=w314:cluster{string[]})  [unwired: 1 in]
                n185 = call <vilib>:"NT Read String.vi"("Name"=w317) -> ("String"=w316:string)  [unwired: 9 in, 1 out]
                n186 = Unbundle(w314) -> (w312:string[])
                n187 = Match First String(2:w312, 3:w316) -> (0:w313:i32)  [unwired: 1 out]
                n188 = property on="Test Ring" class="Ring (strict)"("Value"=w313, "Strings []"=w312) -> ()  [unwired: 2 in, 2 out]
                n189 = property on="Test Ring" class="Ring (strict)"("Visible"=TRUE) -> ()  [unwired: 2 in, 2 out]
                n190 = property on="Test Slider" class="Slide (strict)"("Visible"=FALSE) -> ()  [unwired: 2 in, 2 out]
              }
              frame "White Balance  **" {
                n191 = Index Array(array=w323, index=1) -> (element=w324:cluster{string[]})
                n192 = call <vilib>:"NT Read String.vi"("Name"=w326) -> ("String"=w325:string)  [unwired: 9 in, 1 out]
                n193 = Unbundle(w324) -> (w321:string[])
                n194 = Match First String(2:w321, 3:w325) -> (0:w320:i32)  [unwired: 1 out]
                n195 = property on="Test Ring" class="Ring (strict)"("Value"=w320, "Strings []"=w321) -> ()  [unwired: 2 in, 2 out]
                n196 = property on="Test Ring" class="Ring (strict)"("Visible"=TRUE) -> ()  [unwired: 2 in, 2 out]
                n197 = property on="Test Slider" class="Slide (strict)"("Visible"=FALSE) -> ()  [unwired: 2 in, 2 out]
              }
              frame "Exposure  **" {
                n198 = Index Array(array=w332, index=2) -> (element=w333:cluster{string[]})
                n199 = call <vilib>:"NT Read String.vi"("Name"=w335) -> ("String"=w334:string)  [unwired: 9 in, 1 out]
                n200 = Unbundle(w333) -> (w329:string[])
                n201 = Match First String(2:w329, 3:w334) -> (0:w330:i32)  [unwired: 1 out]
                n202 = property on="Test Ring" class="Ring (strict)"("Value"=w330, "Strings []"=w329) -> ()  [unwired: 2 in, 2 out]
                n203 = property on="Test Ring" class="Ring (strict)"("Visible"=TRUE) -> ()  [unwired: 2 in, 2 out]
                n204 = property on="Test Slider" class="Slide (strict)"("Visible"=FALSE) -> ()  [unwired: 2 in, 2 out]
              }
              frame "Exposure Priority  **" {
                n205 = Index Array(array=w341, index=3) -> (element=w342:cluster{string[]})
                n206 = call <vilib>:"NT Read String.vi"("Name"=w344) -> ("String"=w343:string)  [unwired: 9 in, 1 out]
                n207 = Unbundle(w342) -> (w338:string[])
                n208 = Match First String(2:w338, 3:w343) -> (0:w339:i32)  [unwired: 1 out]
                n209 = property on="Test Ring" class="Ring (strict)"("Value"=w339, "Strings []"=w338) -> ()  [unwired: 2 in, 2 out]
                n210 = property on="Test Ring" class="Ring (strict)"("Visible"=TRUE) -> ()  [unwired: 2 in, 2 out]
                n211 = property on="Test Slider" class="Slide (strict)"("Visible"=FALSE) -> ()  [unwired: 2 in, 2 out]
              }
              frame "Color Enable  **" {
                n212 = Index Array(array=w350, index=4) -> (element=w351:cluster{string[]})
                n213 = call <vilib>:"NT Read String.vi"("Name"=w353) -> ("String"=w352:string)  [unwired: 9 in, 1 out]
                n214 = Unbundle(w351) -> (w347:string[])
                n215 = Match First String(2:w347, 3:w352) -> (0:w348:i32)  [unwired: 1 out]
                n216 = property on="Test Ring" class="Ring (strict)"("Value"=w348, "Strings []"=w347) -> ()  [unwired: 2 in, 2 out]
                n217 = property on="Test Ring" class="Ring (strict)"("Visible"=TRUE) -> ()  [unwired: 2 in, 2 out]
                n218 = property on="Test Slider" class="Slide (strict)"("Visible"=FALSE) -> ()  [unwired: 2 in, 2 out]
              }
              frame Default {
                n219 = property on="Test Ring" class="Ring (strict)"("Visible"=FALSE) -> ()  [unwired: 2 in, 2 out]
                n220 = property on="Test Slider" class="Slide (strict)"("Visible"=FALSE) -> ()  [unwired: 2 in, 2 out]
              }
              frame "Brightness  **", "Color Level  **", "Compression  **", "FPS  **", "Sharpness  **" {
                n221 = call <vilib>:"NT Read Number.vi"("Name"=w359) -> ("Numeric"=w358:dbl)  [unwired: 9 in, 1 out]
                n222 = local write "Test Slider"(w358) -> ()
                n223 = property on="Test Slider" class="Slide (strict)"("Visible"=TRUE, "Scale.Maximum"=100.0 ("Scale.Range:Maximum")) -> ()  [unwired: 2 in, 2 out]
                n224 = property on="Test Ring" class="Ring (strict)"("Visible"=FALSE) -> ()  [unwired: 2 in, 2 out]
              }
            }
          }
        }
        n225 = property on="Progress" class="Clust (strict)"("Visible"=FALSE) -> ()  [unwired: 2 in, 2 out]
      }
      event "Test Name": Mouse Enter {
        # "Populate the ring with the list of tests"
        n226 = event-data() -> ()  [unwired: 1 in, 1 out]
        n227 = call <vilib>:"NT Read String Array.vi"("Name"="/TestMode/TestList") -> ("String Array"=w367:string[])  [unwired: 9 in, 1 out]
        n228 = Build Array (concatenate)("Select the test to run...", w367) -> (w366:string[])
        n229 = property on="Test Name" class="Ring (strict)"("Strings []"=w366) -> ()  [unwired: 2 in, 2 out]
      }
      event "Test Name": Value Change {
        w369 = FALSE ("Visible")
        # "Tell the robot the test name to run"
        n230 = event-data() -> ("NewVal"=w373:u16)  [unwired: 1 in]
        n231 = property on="Test Name" class="Ring (strict)"() -> ("Strings []"=w374:string[])  [unwired: 2 in, 2 out]
        n232 = local write "Progress"(T6 {"Test Progress"=0, "Test Progress Text"=""} ("Progress")) -> ()
        n233 = Index Array(array=w374, index=w373) -> (element=w372:string)
        n234 = call <vilib>:"NT Write String.vi"("String"=w372, "Name"="/TestMode/TestName") -> ()  [unwired: 9 in, 1 out]
        n235 = property on="Progress" class="Clust (strict)"("Visible"=TRUE) -> ()  [unwired: 2 in, 2 out]
        n236 = property on="Motor" class="Clust (strict)"("Visible"=w369) -> ()  [unwired: 2 in, 2 out]
        n237 = property on="Test Slider" class="Slide (strict)"("Visible"=w369) -> ()  [unwired: 2 in, 2 out]
        n238 = property on="On/Off" class="Bool (strict)"("Visible"=w369) -> ()  [unwired: 2 in, 2 out]
        n239 = property on="Rev/Fwd" class="Clust (strict)"("Visible"=w369) -> ()  [unwired: 2 in, 2 out]
        n240 = property on="Test Ring" class="Ring (strict)"("Visible"=w369) -> ()  [unwired: 2 in, 2 out]
      }
      event "Select Auto": Mouse Enter {
        # "Populate the combo box with the list of autonomous options"
        n241 = event-data() -> ()  [unwired: 1 in, 1 out]
        n242 = call <vilib>:"NT Read String Array.vi"("Name"="Auto List") -> ("String Array"=w376:string[])  [unwired: 9 in, 1 out]
        n243 = property on="Select Auto" class="CmbBox"("Strings[]"=w376) -> ()  [unwired: 2 in, 2 out]
      }
      event "Select Auto": Value Change {
        # "User modified the Auto Selection. Write to NT variable so robot knows."
        n244 = event-data() -> ("NewVal"=w379:string)  [unwired: 1 in]
        n245 = call <vilib>:"NT Write String.vi"("String"=w379, "Name"="Auto Selector") -> ()  [unwired: 9 in, 1 out]
      }
      event "Command Selection": Value Change {
        # "Get the params and show in table"
        n246 = event-data() -> ("NewVal"=w385:i32)  [unwired: 1 in]
        n247 = property on="Command Selection" class="MCListbox (strict)"() -> ("ItemNames"=w383:string[][])  [unwired: 2 in, 2 out]
        n248 = call <vilib>:"WPI_DashboardUpdate Command Params.vi"("NewVal"=w385, "Commands"=w383, "Param Tbl"=w384) -> ()  [unwired: 8 in, 1 out]
      }
      event "Execute Command": Value Change {
        # "Started one, Unique ID holds\nresponse"
        n249 = event-data() -> ()  [unwired: 1 in, 1 out]
        n250 = property on="Command Selection" class="MCListbox (strict)"() -> ("ItemNames"=w396:string[][])  [unwired: 2 in, 2 out]
        n251 = Index Array(array=w396, index (row)="Command Selection", index (col)=0) -> (element=w394:string)
        n252 = call <vilib>:"Invoke Commands.vi"("Command Params"="Command Params", "Function Name"=w394) -> ("Params"=w390:u8, "Started"=w389:bool)  [unwired: 7 in, 1 out]
        n253 = Array Subset(array="Command Params", length (row)=w390) -> (w391:string[][])  [unwired: 3 in]
        n254 = Select(t="Executing" ("Cmd Status"), s=w389, f="" ("Cmd Status")) -> (s? t:f=→"Cmd Status":string)
      }
      event "Command Selection": Double Click {
        n255 = event-data() -> ("Row"=w404:i32)  [unwired: 1 in]
        n256 = property on="Command Selection" class="MCListbox (strict)"() -> ("ItemNames"=w407:string[][])  [unwired: 2 in, 2 out]
        n257 = local read "Command Params"() -> (w403:string[][])
        n258 = Index Array(array=w407, index (row)=w404, index (col)=0) -> (element=w405:string)
        n259 = call <vilib>:"Invoke Commands.vi"("Command Params"=w403, "Function Name"=w405) -> ("Params"=w402:u8, "Started"=w397:bool)  [unwired: 7 in, 1 out]
        n260 = Array Subset(array=w403, length (row)=w402) -> (w401:string[][])  [unwired: 3 in]
        n261 = Select(t="Executing" ("Cmd Status"), s=w397, f="" ("Cmd Status")) -> (s? t:f=w398:string)
        n262 = local write "Cmd Status"(w398) -> ()
      }
      event "CheckList": Double Click {
        # "Shift clears all"
        # "Update symbols on the listbox"
        n263 = event-data() -> ("PlatMods.Shift"=w409:bool, "Row"=w411:i32)  [unwired: 1 in]
        n264 = case shown="True" w409 {
          tunnel: w411 -> [w415 _]
          tunnel: 1 -> [w414 _]
          frame False {
            n265 = property on="CheckList" class="LstBox (strict)"() -> ("Item Symbols"=w413:i32[])  [unwired: 2 in, 2 out]
            n266 = Replace Array Subset(array=w413, new element=w414, index=w415) -> (w412:i32[])
            n267 = property on="CheckList" class="LstBox (strict)"("Item Symbols"=w412) -> ()  [unwired: 2 in, 2 out]
          }
          frame True {
            w416 = 0 ("Top Row")
            n268 = property on="CheckList" class="LstBox (strict)"() -> ("Number of Rows"=w418:u32)  [unwired: 2 in, 2 out]
            n269 = Initialize Array(0, w418) -> (w417:i32[])
            n270 = property on="CheckList" class="LstBox (strict)"("Top Row"=w416, "Value"=w416, "Item Symbols"=w417) -> ()  [unwired: 2 in, 2 out]
          }
        }
      }
      event "CheckList": Key Down {
        # "Update symbols on the listbox\nLeft and right keys check and uncheck"
        n271 = event-data() -> ("VKey"=w422:T20)  [unwired: 1 in]
        n272 = case shown="\"Left\", \"Right\"" w422 {
          selector: w422 -> [w427 _]
          tunnel: eventvkey."Left" ("VKey") -> [w425 _]
          frame "Left", "Right" {
            n273 = Equal?(x=w425, y=w427) -> (x = y?=w426:bool)
            n274 = Select(t=0, s=w426, f=1) -> (s? t:f=w428:i32)
            n275 = property on="CheckList" class="LstBox (strict)"() -> ("Item Symbols"=w431:i32[])  [unwired: 2 in, 2 out]
            n276 = Replace Array Subset(array=w431, new element=w428, index="CheckList") -> (w430:i32[])
            n277 = property on="CheckList" class="LstBox (strict)"("Item Symbols"=w430) -> ()  [unwired: 2 in, 2 out]
          }
          frame Default {
          }
        }
      }
      event "Motor.Enable": Value Change {
        # "When the test mode otor enable helper is set, update that\ntree row item's value"
        n278 = event-data() -> ("NewVal"=w437:bool)  [unwired: 1 in]
        n279 = Unbundle("Motor") -> ("Value"=w436:dbl)  [unwired: 1 out]
        n280 = Select(t=w436, s=w437, f=0.0) -> (s? t:f=w434:dbl)
        n281 = call <vilib>:"NT Write Number.vi"("Numeric"=w434, "Name"=w433) -> ()  [unwired: 9 in, 1 out]
      }
      event "Test Slider": Value Change {
        # "When the test mode slider helper is set, update that\ntree row item's value"
        n282 = event-data() -> ("NewVal"=w440:dbl)  [unwired: 1 in]
        n283 = call <vilib>:"NT Write Number.vi"("Numeric"=w440, "Name"=w441) -> ()  [unwired: 9 in, 1 out]
      }
      event "On/Off": Value Change {
        # "When the test mode on/off helper value is set, update that\ntree row item's value"
        n284 = event-data() -> ("NewVal"=w445:bool)  [unwired: 1 in]
        n285 = Boolean To (0,1)(Boolean=w445) -> (0, 1=w444:i16)
        n286 = call <vilib>:"NT Write Number.vi"("Numeric"=w444, "Name"=w443) -> ()  [unwired: 9 in, 1 out]
      }
      event "Rev/Fwd": Value Change {
        # "When the test mode helper value for relays is set, update that\ntree row item's value"
        n287 = event-data() -> ("NewVal.Forward"=w453:bool, "NewVal.Reverse"=w452:bool)  [unwired: 1 in]
        n288 = Boolean To (0,1)(Boolean=w453) -> (0, 1=w449:i16)
        n289 = Boolean To (0,1)(Boolean=w452) -> (0, 1=w451:i16)
        n290 = Negate(x=w451) -> (-x=w450:i16)
        n291 = Add(x=w449, y=w450) -> (x+y=w448:i16)
        n292 = call <vilib>:"NT Write Number.vi"("Numeric"=w448, "Name"=w447) -> ()  [unwired: 9 in, 1 out]
      }
      event "Test Ring": Value Change {
        # "When a test mode helper value is selected from the ring,\nset the tree item's variable to the string value"
        n293 = event-data() -> ("NewVal"=w457:u16)  [unwired: 1 in]
        n294 = property on="Test Ring" class="Ring (strict)"() -> ("Strings []"=w458:string[])  [unwired: 2 in, 2 out]
        n295 = Index Array(array=w458, index=w457) -> (element=w456:string)
        n296 = call <vilib>:"NT Write String.vi"("String"=w456, "Name"=w455) -> ()  [unwired: 9 in, 1 out]
      }
      event "Rec Mode": Value Change {
        # "Update globals for recording mode and path to read log from.\nClear when logging and let NetworkTables set path for vision to\nuse."
        n297 = event-data() -> ("NewVal"=w469:enum32{"Stop", "Record", "Playback"})  [unwired: 1 in]
        n298 = global write "WPI_DashboardLogging Global.vi" "Logging Filename"(path "") -> ()
        n299 = global write "WPI_DashboardLogging Global.vi" "Recording"(w469) -> ()
        n300 = case shown="\"Playback\"" w469 {
          tunnel: w468 -> [_ w471 w480]
          tunnel: [_ _ w479] -> w466
          tunnel: [_ _ w478] -> _
          tunnel: w464 -> [_ _ w476]
          tunnel: cluster{i32, i32} {-250, 170} -> [_ _ w475]
          tunnel: [_ _ T21 {"Image Size"=TRUE, "Image Type"=TRUE, "Pixel Value"=TRUE, "ROI Information"=TRUE, "Zoom Factor"=FALSE} ("Image Information Shown:All Elements")] -> w462
          tunnel: [_ _ TRUE ("Zoom Factor")] -> w461
          tunnel: w460 -> [_ _ w472]
          frame Default {
          }
          frame "Stop", "Record" {
            # "Place Window too"
            n301 = invoke class="VI" method="FP.Close"(reference=w471) -> (reference out=w470:refnum<vi>)  [unwired: 2 in, 2 out]
            n302 = invoke class="VI" method="Abort VI"(reference=w470) -> ()  [unwired: 2 in, 3 out]
          }
          frame "Playback" {
            n303 = call "Open Playback Panel.vi"("Offset"=w475, "DB VI Ref"=w476, "Playback in"=w480) -> ("Playback out"=w477:refnum<vi>)  [unwired: 8 in]
            n304 = register-events(w477, w472) -> (reference out=w479:refnum<event-registration>, error out=w478:errorcluster)  [unwired: 2 in]
          }
        }
        n305 = property on="Camera Image" class="ImageControl"("Image Information Shown"=w462, "Image Information Visible"=w461) -> ()  [unwired: 2 in, 2 out]
        n306 = call <vilib>:"WPI_DashboardNT Log FieldName Cache.vi"("Operation"=enum16{"Lookup/Add", "Index", "Clear"}."Clear") -> ()  [unwired: 8 in, 3 out]
      }
      event Panel Close {
        w482 = enum32{"Stop", "Record", "Playback"}."Stop" ("Rec Mode")
        # "Playback window has been closed, abort"
        n307 = event-data() -> ()  [unwired: 1 in, 4 out]
        n308 = local write "Rec Mode"(w482) -> ()
        n309 = global write "WPI_DashboardLogging Global.vi" "Recording"(w482) -> ()
      }
      event Panel Close {
        # "Abort playback window and ourself"
        n310 = event-data() -> ()  [unwired: 1 in, 4 out]
        n311 = invoke class="VI" method="FP.Close"(reference=w486) -> (reference out=w485:refnum<vi>)  [unwired: 2 in, 2 out]
        n312 = invoke class="VI" method="Abort VI"(reference=w485) -> (error out=w484:errorcluster)  [unwired: 2 in, 2 out]
        n313 = invoke class="VI" method="Abort VI"(error in=w484) -> ()  [unwired: 2 in, 3 out]
      }
      event User Event {
        n314 = event-data() -> ("IDs"=w493:cluster{"RPC field ID":u16, "Unique ID":u16}, "String"=w492:string)  [unwired: 1 in]
        n315 = Bundle("IDs"=w493, "String"=w492) -> (w491:T8)  [unwired: 1 in]
        n316 = call <vilib>:"Retrieve RPC Response.vi"("RPC Response"=w491) -> ("Output"=w489:string[][])  [unwired: 10 in]
        n317 = Build Array (concatenate)(w487, w489) -> (w488:string[][])
        n318 = local write "Command Params"(w488) -> ()
        n319 = local write "Cmd Status"("" ("Cmd Status")) -> ()
      }
      event "Tree": Double Click {
        n320 = event-data() -> ("PlatMods"=w497:T24, "Tag"=w496:string)  [unwired: 1 in]
        n321 = Unbundle(w497) -> ("Shift"=w495:bool)  [unwired: 4 out]
        n322 = Not(x=w495) -> (.not. x?=w494:bool)
        n323 = call <vilib>:"NT Update Persistence.vi"("Persistence"=w494, "Name"=w496) -> ()  [unwired: 9 in, 1 out]
      }
    }
  }
  n324 = while {
    tunnel: w68 -> [w500]
    i -> [w503]
    stop <- FALSE stop-if-true
    n325 = Wait (ms)(milliseconds to wait=u32 100) -> ()  [unwired: 1 out]
    n326 = case shown="\"Playback\"" "Rec Mode" {
      tunnel: w503 -> [_ _ w518]
      tunnel: [u32 2829099 ("Base Color") u32 11141120 ("Target Color") w507] -> w499
      frame "Stop", Default {
        # "Reset the color, extra updates don't cost much"
      }
      frame "Record" {
      }
      frame "Playback" {
        # "Playback"
        n327 = Quotient & Remainder(x=w518, y=u32 50 ("milliseconds to wait")) -> (x-y*floor(x/y)=w514:u32)  [unwired: 1 out]
        n328 = Divide(x=w514, y=u32 50 ("milliseconds to wait")) -> (x/y=w511:dbl)
        n329 = Multiply(x=6.283185307179586, y=w511) -> (x*y=w516:dbl)
        n330 = Sine(x=w516) -> (sin(x)=w515:dbl)
        n331 = Absolute Value(x=w515) -> (abs(x)=w508:dbl)
        n332 = call "Interpolate RGB Color.vi"("Proportion"=w508, "Target Color"=u32 30976, "Base Color"=u32 2829099) -> ("Result Color"=w507:u32)  [unwired: 8 in]
      }
    }
    n333 = property class="Pane"(reference=w500, "PaneColor"=w499) -> ()  [unwired: 1 in, 2 out]
  }
  n334 = local write "Dashboard Tab"(T2."Drive" ("Dashboard Tab")) -> ()
  n335 = property on="On/Off" class="Bool (strict)"("Visible"=w39) -> ()  [unwired: 2 in, 2 out]
  n336 = property on="Motor" class="Clust (strict)"("Visible"=w39) -> ()  [unwired: 2 in, 2 out]
  n337 = property on="Progress" class="Clust (strict)"("Visible"=w39) -> ()  [unwired: 2 in, 2 out]
  n338 = property on="Test Ring" class="Ring (strict)"("Visible"=w39) -> ()  [unwired: 2 in, 2 out]
  n339 = property on="Rev/Fwd" class="Clust (strict)"("Visible"=w39) -> ()  [unwired: 2 in, 2 out]
  n340 = while {
    tunnel: u16 1741 ("timeout ms (25000)") -> [w520]
    stop <- FALSE stop-if-true
    n341 = TCP Create Listener(10:w520) -> (0:w519:errorcluster, 3:w521:refnum<k5>)  [unwired: 4 in, 1 out]
    n342 = case shown="No Error" w519 {
      selector: w519 -> [w523 _]
      tunnel: w521 -> [w524 _]
      frame No Error {
        n343 = while {
          tunnel: w524 -> [w527]
          tunnel: w523 -> [w526]
          stop <- FALSE stop-if-true
          n344 = TCP Wait On Listener(8:w526, 11:w527) -> (0:w528:errorcluster, 4:w529:refnum<k5>)  [unwired: 2 in, 3 out]
          n345 = local write "TCP"(w529) -> ()
          n346 = case shown="No Error" w528 {
            frame No Error {
            }
            frame Error {
              n347 = Wait (ms)(milliseconds to wait=u32 1000) -> ()  [unwired: 1 out]
            }
          }
        }
      }
      frame Error {
        n348 = Wait (ms)(milliseconds to wait=u32 1000) -> ()  [unwired: 1 out]
      }
    }
  }
  n349 = local write "Command Selection"(u16 0 ("milliseconds to wait")) -> ()
  n350 = local write "Command Params"(string[][] [] ("Command Params")) -> ()
  n351 = global write "WPI_DashboardLogging Global.vi" "Recording"(w62) -> ()
  n352 = local write "Rec Mode"(w62) -> ()
  n353 = call <vilib>:"NT Write String.vi"("String"="Select Auto", "Name"="Auto Selector") -> ()  [unwired: 9 in, 1 out]
